vi "数据查询_仪器日志.vi"() -> ()   [LabVIEW 2016]
uses:
  <vilib>/Utility/miscctls.llb/LVRowAndColumnUnsignedTypeDef.ctl
  <vilib>/Utility/miscctls.llb/LVPositionTypeDef.ctl
  <vilib>/Utility/miscctls.llb/LVPointTypeDef.ctl
  <userlib>/_OpenG.lib/array/array.llb/Sort 2D Array (String)__ogtk.vi
  <userlib>/_OpenG.lib/array/array.llb/Sort 1D Array (I32)__ogtk.vi
panel:
  in  "触发查询":bool
  out "显示项":string[](array[string])
  out "确定查询":bool
  out "condition":string
  in  "数据列表选择框":string(xcontrol)
  in  "导出":bool
  in  "条件筛选":bool
  in  "数据表":T1
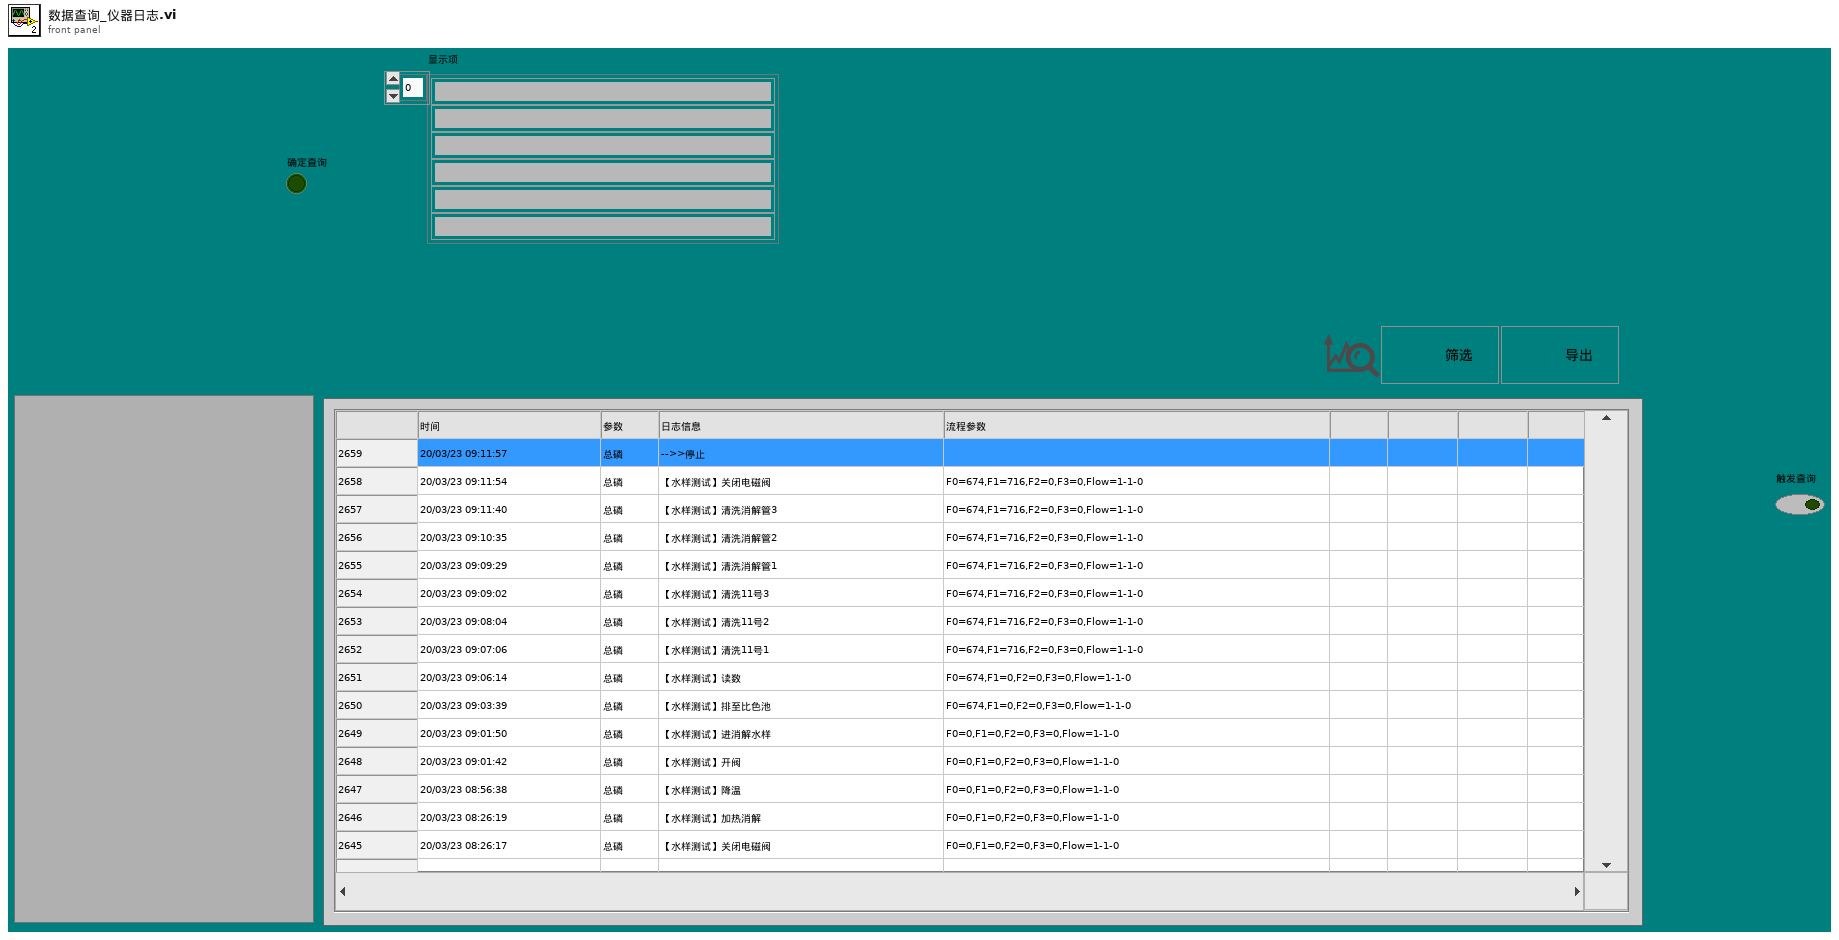
[diagram p1: front panel]
types:
  T1 = typedef "数据查询大列表框.ctl" = i32
  T2 = typedef "LVPositionTypeDef.ctl" = cluster{"Left":i32, "Top":i32}
  T3 = typedef "LVRowAndColumnUnsignedTypeDef.ctl" = cluster{"Row":u32, "Column":u32}
  T4 = typedef "LVPointTypeDef.ctl" = cluster{"Horizontal":i16, "Vertical":i16}
  T5 = enum8{"Enabled", "Disabled", "Disabled and Grayed Out"}
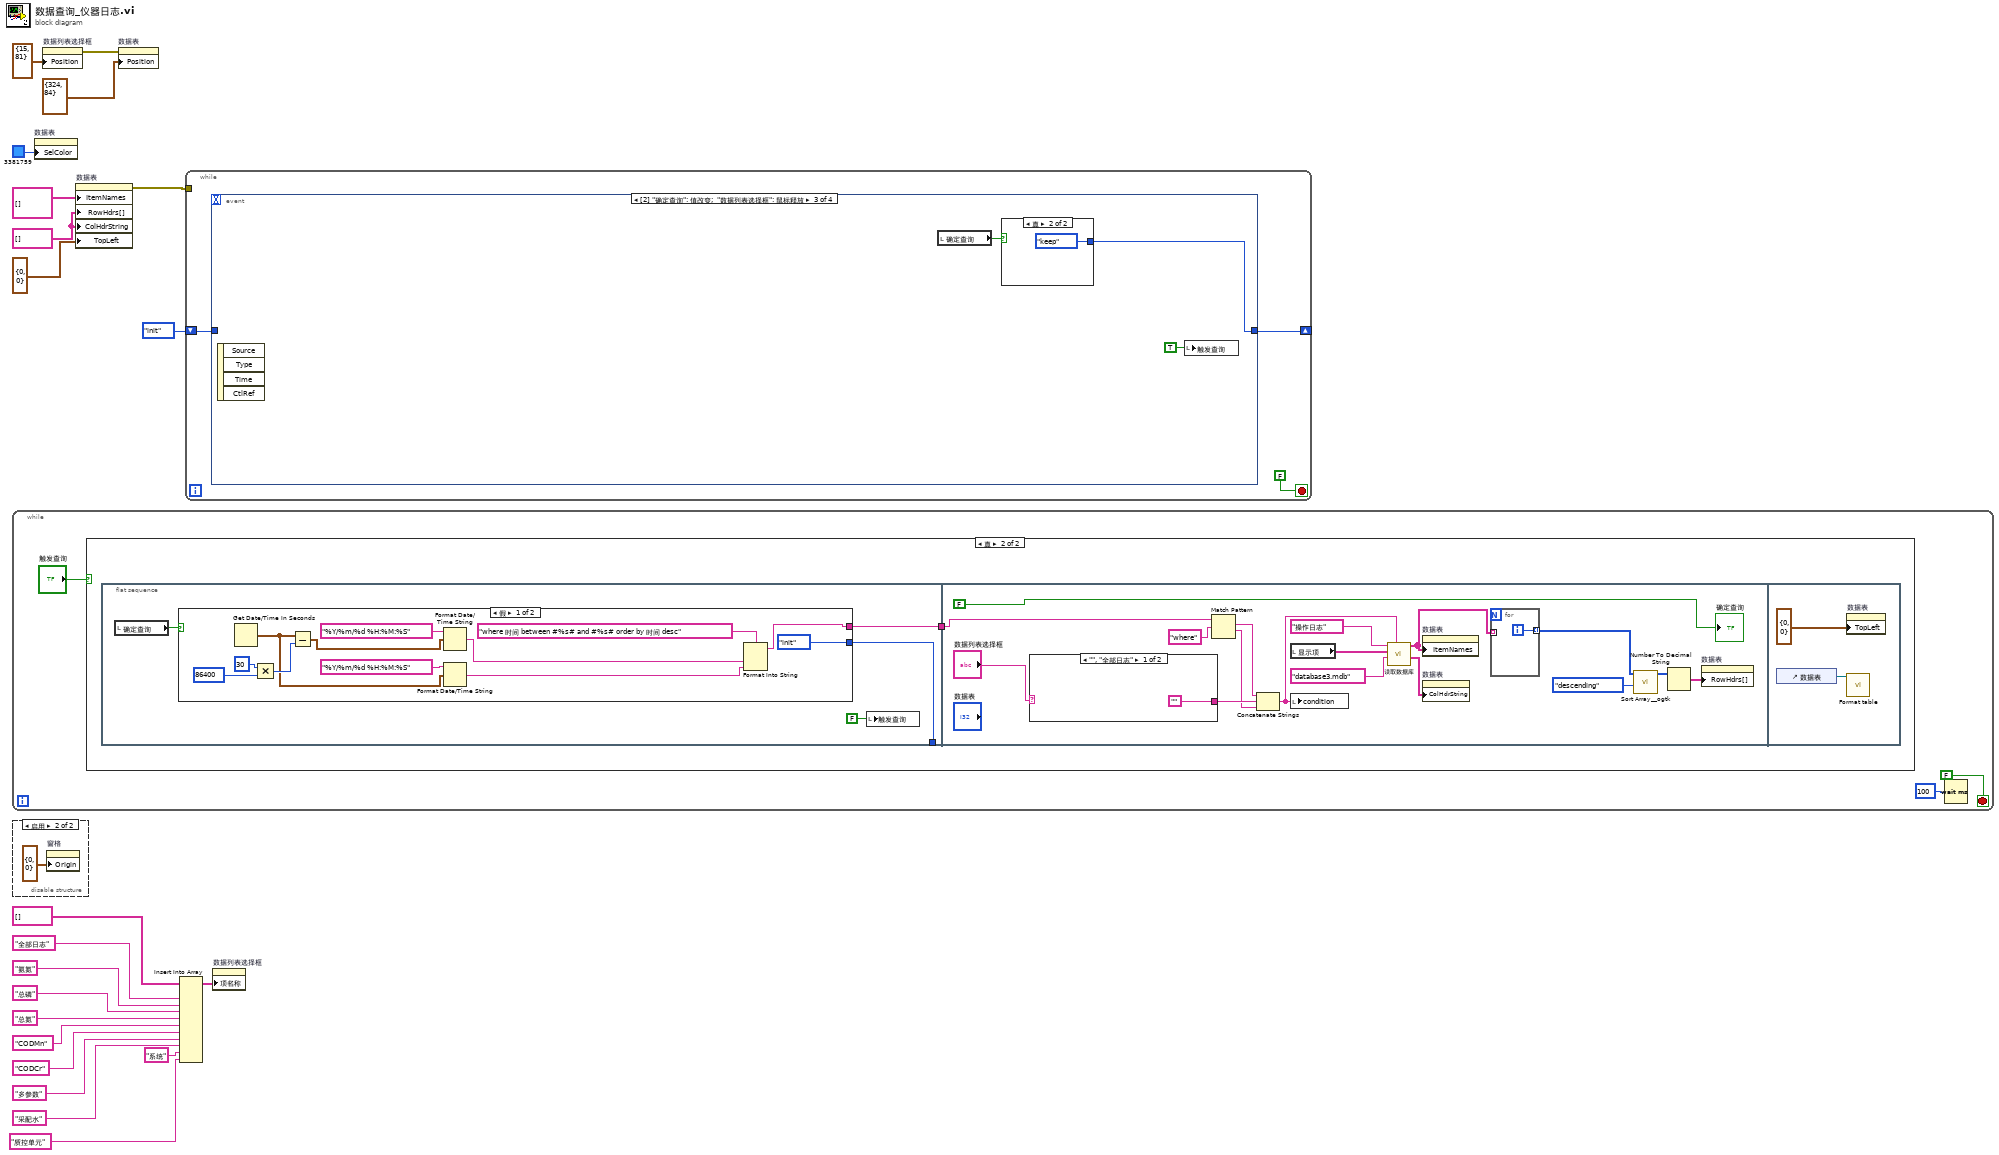
[diagram p0: block diagram]
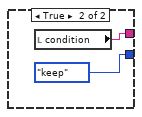
[diagram p3: hidden frame]
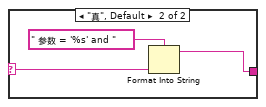
[diagram p4: hidden frame]
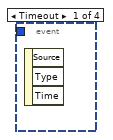
[diagram p5: hidden frame]
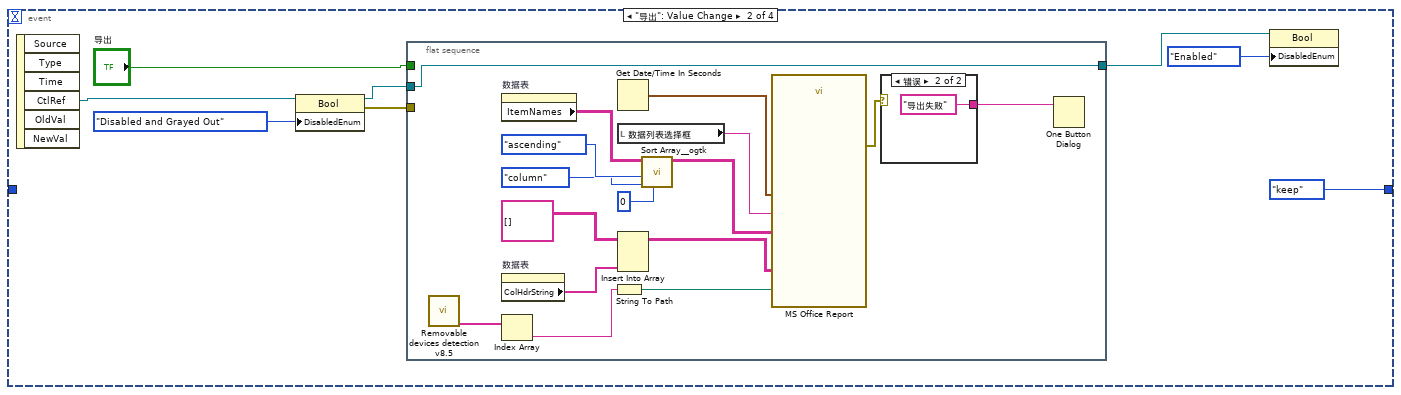
[diagram p6: hidden frame]
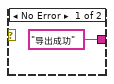
[diagram p7: hidden frame]
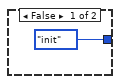
[diagram p8: hidden frame]
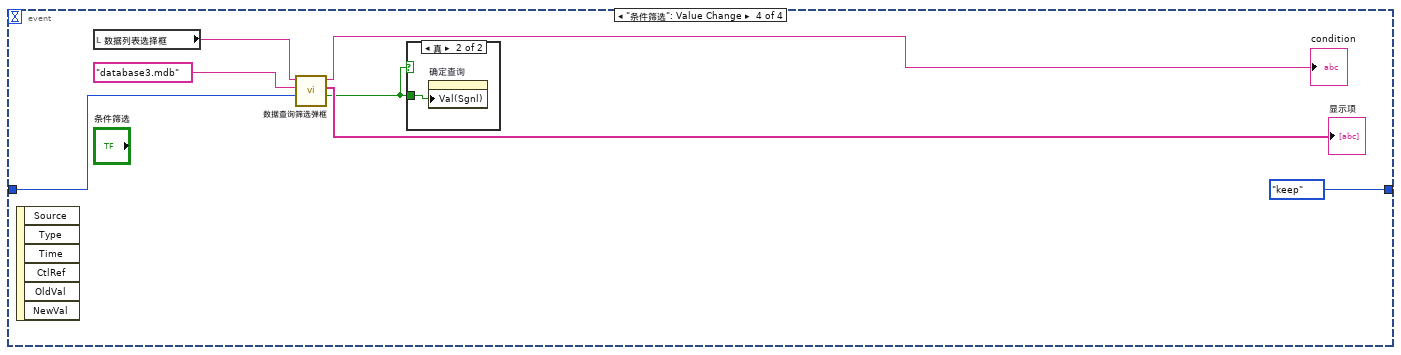
[diagram p9: hidden frame]
diagram:
  w9 = string[] [] ("行首字符串[]")
  n1 = while {
    stop <- FALSE stop-if-true
    n2 = case shown="真" "触发查询" {
      frame False {
      }
      frame True {
        n3 = flat-sequence {
          tunnel: [w28] -> w25
          tunnel: [w27] -> _
          tunnel: w25 -> [w49]
          frame #0 {
            n4 = local read "确定查询"() -> (w29:bool)
            n5 = case shown="假" w29 {
              tunnel: [w32 w42] -> w28
              tunnel: [enum16{"init", "keep"}."init" ("是否初始化") enum16{"init", "keep"}."keep" ("是否初始化")] -> w27
              frame False {
                n6 = Get Date/Time In Seconds() -> (seconds since 1Jan1904=w30:timestamp)
                n7 = Multiply(x=30, y=86400) -> (x*y=w33:i32)
                n8 = Subtract(x=w30, y=w33) -> (x-y=w38:timestamp)
                n9 = Format Date/Time String(time format string (%c)="%Y/%m/%d %H:%M:%S" ("时间格式字符串(%c)"), seconds (now)=w38) -> (date/time string=w40:string)  [unwired: 1 in]
                n10 = Format Date/Time String(time format string (%c)="%Y/%m/%d %H:%M:%S" ("时间格式字符串(%c)"), seconds (now)=w30) -> (date/time string=w41:string)  [unwired: 1 in]
                n11 = Format Into String(format string="where 时间 between #%s# and #%s# order by 时间 desc", w40, w41) -> (resulting string=w32:string)  [unwired: 2 in, 1 out]
              }
              frame True {
                n12 = local read "condition"() -> (w42:string)
              }
            }
            n13 = local write "触发查询"(FALSE ("触发查询")) -> ()
          }
          frame #1 {
            n14 = case shown="\"\", \"全部日志\"" "数据列表选择框" {
              selector: "数据列表选择框" -> [_ w63]
              tunnel: ["" w62] -> w46
              frame "", "全部日志" {
              }
              frame "真", Default {
                n15 = Format Into String(format string=" 参数 = '%s' and " ("condition"), w63) -> (resulting string=w62:string)  [unwired: 2 in, 1 out]
              }
            }
            n16 = Match Pattern(string=w49, regular expression="where") -> (match substring=w47:string, after substring=w45:string)  [unwired: 1 in, 2 out]
            n17 = Concatenate Strings(w47, w46, w45) -> (w44:string)
            n18 = local read "显示项"() -> (w51:string[])
            n19 = local write "condition"(w44) -> ()
            n20 = call "读取数据库.vi"("condition"=w44, "database"="database3.mdb", "显示项"=w51, "组合框"="操作日志") -> ("columns"=w60:string[], "表格"=w53:string[][])  [unwired: 4 in, 2 out]
            n21 = property on="数据表" class="MCListbox (严格)"("ItemNames"=w53) -> ()  [unwired: 2 in, 2 out]
            n22 = property on="数据表" class="MCListbox (严格)"("ColHdrString"=w60) -> ()  [unwired: 2 in, 2 out]
            n23 = for {
              tunnel: w53 -> [_] mode=indexing
              tunnel: [w65] -> w58 mode=indexing
              i -> [w65]
            }
            n24 = call-poly <userlib>:"Sort Array__ogtk.vi"("Order"=enum16{"ascending", "descending"}."descending", "Array in"=w58) -> ("Sorted Array out"=w55:i32[])  [unwired: 8 in, 1 out]
            n25 = Number To Decimal String(number=w55) -> (decimal integer string=w57:string[])  [unwired: 1 in]
            n26 = property on="数据表" class="MCListbox (严格)"("RowHdrs[]"=w57) -> ()  [unwired: 2 in, 2 out]
            "确定查询" <- FALSE ("确定查询")
          }
          frame #2 {
            n27 = control-ref of="数据表"() -> (w66:refnum<vi>)
            n28 = property on="数据表" class="MCListbox (严格)"("TopLeft"=T3 {"Row"=0, "Column"=0} ("索引值")) -> ()  [unwired: 2 in, 2 out]
            n29 = call "Format table.vi"("Table输入"=w66) -> ()  [unwired: 11 in]
          }
        }
      }
    }
    n30 = Wait (ms)(milliseconds to wait=u32 100 ("等待时间（毫秒）")) -> ()  [unwired: 1 out]
  }
  n31 = disable-structure shown="启用" {
    frame Disabled {
    }
    frame Enabled {
      n32 = property on="窗格" class="Pane"("Origin"=T4 {"Horizontal"=0, "Vertical"=0} ("原点")) -> ()  [unwired: 2 in, 2 out]
    }
  }
  n33 = property on="数据表" class="MCListbox (严格)"("SelColor"=u32 3381759) -> ()  [unwired: 2 in, 2 out]
  n34 = property on="数据列表选择框" class="数据列表选择框 (严格)"("Position"=T2 {"Left"=15, "Top"=81} ("位置")) -> (error out=w2:errorcluster)  [unwired: 2 in, 1 out]
  n35 = property on="数据表" class="MCListbox (严格)"("ItemNames"=string[][] [] ("项名"), "RowHdrs[]"=w9, "ColHdrString"=w9, "TopLeft"=T3 {"Row"=0, "Column"=0} ("左上可见单元格")) -> (error out=w11:errorcluster)  [unwired: 2 in, 1 out]
  n36 = property on="数据表" class="MCListbox (严格)"(error in=w2, "Position"=T2 {"Left"=324, "Top"=84} ("位置")) -> ()  [unwired: 1 in, 2 out]
  n37 = Insert Into Array(array=string[] [], new element #1="全部日志" ("新元素/子数组"), new element #2="氨氮" ("新元素/子数组"), new element #3="总磷" ("新元素/子数组"), new element #4="总氮" ("新元素/子数组"), new element #5="CODMn" ("新元素/子数组"), new element #6="CODCr" ("新元素/子数组"), new element #7="多参数" ("新元素/子数组"), new element #8="采配水" ("新元素/子数组"), new element #9="系统" ("新元素/子数组"), new element #10="质控单元" ("新元素/子数组")) -> (w7:string[])  [unwired: 1 in]
  n38 = while {
    tunnel: w11 -> [_]
    shift-right: [w69] -> _
    shift-left: enum16{"init", "keep"}."init" ("是否初始化") -> [w70]
    stop <- FALSE stop-if-true
    n39 = event shown="[2] \"确定查询\": 值改变;  \"数据列表选择框\": 鼠标释放" {
      selector: _ -> [_ _ _ _]
      dyn-events: _ -> [_ _ _ _]
      timeout: _ -> [_ _ _ _]
      tunnel: w70 -> [_ _ _ w107]
      tunnel: [_ enum16{"init", "keep"}."keep" ("是否初始化") w99 enum16{"init", "keep"}."keep" ("是否初始化")] -> w69
      event Timeout {
        n40 = event-data() -> ()  [unwired: 1 in, 3 out]
      }
      event "导出": Value Change {
        n41 = event-data() -> ("CtlRef"=w73:refnum<vi>)  [unwired: 1 in, 5 out]
        n42 = property class="Bool"(reference=w73, "DisabledEnum"=T5."Disabled and Grayed Out" ("禁用")) -> (reference out=w77:refnum<vi>, error out=w78:errorcluster)  [unwired: 1 in]
        n43 = flat-sequence {
          tunnel: w78 -> [_]
          tunnel: [w89] -> w76
          tunnel: w77 -> [w89]
          tunnel: "导出" -> [_]
          frame #0 {
            n44 = call "Removable devices detection v8.5.vi"() -> ("Removable"=w86:string[])  [unwired: 4 out]
            n45 = property on="数据表" class="MCListbox (严格)"() -> ("ItemNames"=w80:string[][])  [unwired: 2 in, 2 out]
            n46 = property on="数据表" class="MCListbox (严格)"() -> ("ColHdrString"=w81:string[])  [unwired: 2 in, 2 out]
            n47 = Index Array(array=w86) -> (element=w85:string)  [unwired: 1 in]
            n48 = String To Path(string=w85) -> (path=w84:path)
            n49 = Get Date/Time In Seconds() -> (seconds since 1Jan1904=w95:timestamp)
            n50 = local read "数据列表选择框"() -> (w90:string)
            n51 = Insert Into Array(array=string[][] [], new element=w81) -> (w82:string[][])  [unwired: 2 in]
            n52 = call-poly <userlib>:"Sort Array__ogtk.vi"("Column/Row to Sort By"=u32 0, "Sort By in"=enum16{"row", "column"}."column", "Order"=enum16{"ascending", "descending"}."ascending", "Array in"=w80) -> ("Sorted Array out"=w94:string[][])  [unwired: 4 in, 3 out]
            n53 = call "MS Office Report"("Path to Save Report"=w84, "导出日期"=w95, "监测参数"=w90, "数据输入"=w94, "字段定义"=w82) -> ("error out"=w88:errorcluster)  [unwired: 21 in, 1 out]
            n54 = case shown="错误" w88 {
              tunnel: ["导出成功" ("消息") "导出失败" ("消息")] -> w87
              frame No Error {
              }
              frame Error {
              }
            }
            n55 = One Button Dialog(message=w87) -> ()  [unwired: 1 in, 1 out]
          }
        }
        n56 = property class="Bool"(reference=w76, "DisabledEnum"=T5."Enabled" ("禁用")) -> ()  [unwired: 1 in, 2 out]
      }
      event "确定查询": Value Change; "数据列表选择框": Mouse Up {
        n57 = event-data() -> ()  [unwired: 1 in, 4 out]
        n58 = local read "确定查询"() -> (w100:bool)
        n59 = case shown="真" w100 {
          tunnel: [enum16{"init", "keep"}."init" ("是否初始化") enum16{"init", "keep"}."keep" ("是否初始化")] -> w99
          frame False {
          }
          frame True {
          }
        }
        n60 = local write "触发查询"(TRUE ("触发查询")) -> ()
      }
      event "条件筛选": Value Change {
        n61 = event-data() -> ()  [unwired: 1 in, 6 out]
        n62 = local read "数据列表选择框"() -> (w108:string)
        n63 = call "数据查询筛选弹框.vi"("是否初始化"=w107, "database"="database3.mdb", "table"=w108) -> ("确定输出"=w104:bool, "显示项"=→"显示项":string[], "condition"=→"condition":string)  [unwired: 5 in, 1 out]
        n64 = case shown="真" w104 {
          tunnel: w104 -> [_ w110]
          frame False {
          }
          frame True {
            n65 = property on="确定查询" class="Bool (严格)"("Val(Sgnl)"=w110) -> ()  [unwired: 2 in, 2 out]
          }
        }
      }
    }
  }
  n66 = property on="数据列表选择框" class="数据列表选择框 (严格)"("项名称"=w7) -> ()  [unwired: 2 in, 2 out]
